vi "Init.vi"(7 "I2C #":T1=-1, 8 "error in (no error)":errorcluster, 10 "Session In":refnum<class "Session.lvclass">) -> (0 "error out":errorcluster, 3 "MCP4018 Digipot Out":refnum<class "MCP4018 Digipot.lvclass">)   [LabVIEW 2020, in "CTI-Peripheral.lvlib" / "MCP4018 Digipot.lvclass"]
uses:
  MCP4018 Digipot.lvclass
  CTI/I2C Connection/I2C Connection.lvclass/I2C Connection.ctl
  MCP4018 Digipot.lvclass/MCP4018 Digipot.ctl
  CTI/I2C Connection/I2C Connection.lvclass
  CTI/I2C Address.ctl
  CTI/CTI.lvlib
  CTI/Session/Session.lvclass
  CTI/I2C Number.ctl
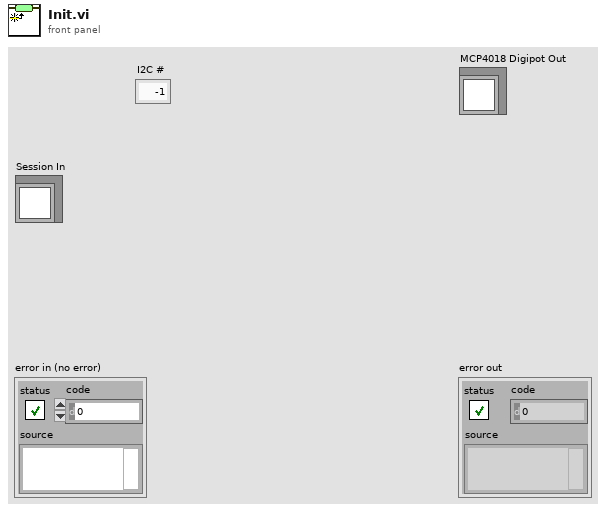
[diagram p1: front panel]
types:
  T1 = typedef "CTI.lvlib/I2C Number.ctl" = i8
  T2 = typedef "CTI.lvlib/I2C Address.ctl" = u8
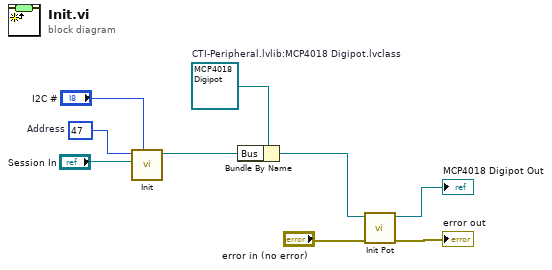
[diagram p0: block diagram]
diagram:
  w5 = refnum<class "MCP4018 Digipot.lvclass"> refnum  # CTI-Peripheral.lvlib:MCP4018 Digipot.lvclass
  w6 = T2 47  # Address
  n1 = call "Init.vi"("I2C #"="I2C #", "Session"="Session In", "Address"=w6) -> ("I2C Connection"=w9:refnum<class "I2C Connection.lvclass">)  [unwired: 7 in, 1 out]
  n2 = Bundle By Name(cluster=w5, "Bus"=w9) -> (w2:refnum<class "MCP4018 Digipot.lvclass">)
  n3 = call "Init Pot.vi"("error in (no error)"="error in (no error)", "MCP4018 Digipot in"=w2) -> ("error out"=→"error out":errorcluster, "MCP4018 Digipot out"=→"MCP4018 Digipot Out":refnum<class "MCP4018 Digipot.lvclass">)  [unwired: 7 in, 1 out]
